vi "Std Dev.vi"(7 "Points":u32=200, 10 "From":refnum<class "Readable.lvclass">) -> (2 "Std Dev.lvclass out":refnum<class "Std Dev.lvclass">)   [LabVIEW 2009, in "Std Dev.lvclass"]
uses:
  Std Dev.lvclass
  Readable/Readable.lvclass
  Std Dev.lvclass/Std Dev.ctl
panel:
  out "error out":errorcluster
  in  "error in (no error)":errorcluster
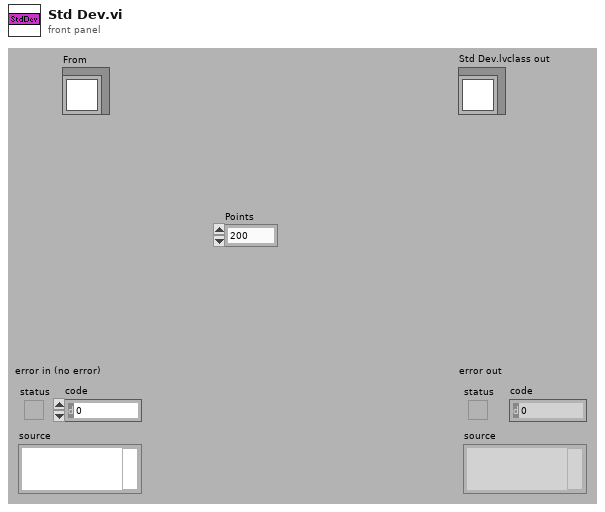
[diagram p1: front panel]
types:
  T1 = typedef "Readable.lvclass/Channel Units.ctl" = string[]
  T2 = typedef "Readable.lvclass/Channel Names.ctl" = string[]
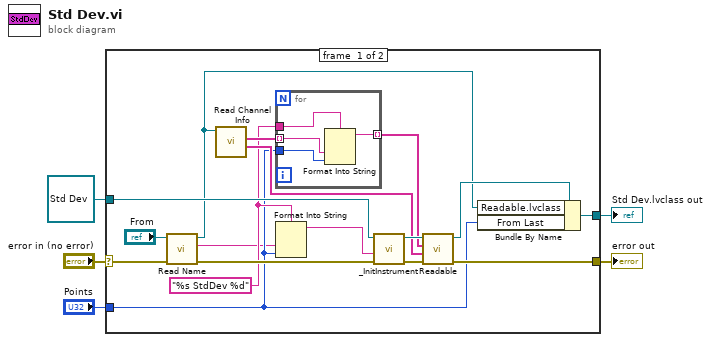
[diagram p0: block diagram]
diagram:
  n1 = case shown="No Error" "error in (no error)" {
    selector: "error in (no error)" -> [w19 w27]
    tunnel: [w13 w27] -> w4
    tunnel: [w22 w28] -> w3
    tunnel: refnum<class "Std Dev.lvclass"> refnum ("Std Dev.lvclass in") -> [w18 w28]
    tunnel: "Points" -> [w7 _]
    frame #0 {
      w8 = "%s StdDev %d" ("format string")
      n2 = call-dynamic "Read Name.vi"("error in (no error)"=w19, "Instrument.lvclass in"="From") -> ("error out"=w20:errorcluster, "Name"=w6:string, "Instrument.lvclass out"=w12:refnum<class "Readable.lvclass">)  [unwired: 7 out]
      n3 = call "Read Channel Info.vi"("Readable.lvclass in"=w12) -> ("Channel Units"=w11:T1, "Channel Names"=w10:T2)  [unwired: 6 in, 3 out]
      n4 = for {
        tunnel: w10 -> [w23] mode=indexing
        tunnel: w7 -> [w24]
        tunnel: [w26] -> w9 mode=indexing
        tunnel: w8 -> [w25]
        n5 = Format Into String(format string=w25, w23, w24) -> (resulting string=w26:string)  [unwired: 2 in, 1 out]
      }
      n6 = Format Into String(format string=w8, w6, w7) -> (resulting string=w16:string)  [unwired: 2 in, 1 out]
      n7 = call-dynamic "_InitInstrument.vi"("error in (no error)"=w20, "Name"=w16, "Instrument in"=w18) -> ("error out"=w14:errorcluster, "Instrument out"=w17:refnum<class "Std Dev.lvclass">)  [unwired: 3 in, 4 out]
      n8 = call "Readable.vi"("error in (no error)"=w14, "Channel Units"=w11, "Channel Names"=w9, "Readable in"=w17) -> ("error out"=w13:errorcluster, "Readable out"=w15:refnum<class "Std Dev.lvclass">)  [unwired: 6 in]
      n9 = Bundle By Name(cluster=w15, "Readable.lvclass"=w12, "From Last"=w7) -> (w22:refnum<class "Std Dev.lvclass">)
    }
    frame #1 {
    }
  }
  "error out" <- w4
  "Std Dev.lvclass out" <- w3
